vi "From.vi"(1 "Value":bool=TRUE) -> (0 "Boolean":refnum<class "Boolean.lvclass">)   [LabVIEW 2018, in "Toolkit.lvlib" / "Data.lvlib" / "Boolean.lvclass"]
uses:
  Boolean.lvclass
  Boolean.lvclass/Boolean.ctl
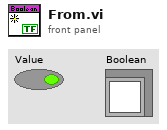
[diagram p1: front panel]
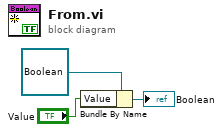
[diagram p0: block diagram]
diagram:
  n1 = Bundle By Name(cluster=refnum<class "Boolean.lvclass"> refnum ("Toolkit.lvlib:Data.lvlib:Boolean.lvclass"), "Value"="Value") -> (→"Boolean":refnum<class "Boolean.lvclass">)
